vi "PicoScope2000UnitInfoSingle.vi"(8 "error in (no error)":errorcluster, 9 "info Enum":i16(ring), 11 "Handle in":i16) -> (0 "error out":errorcluster, 1 "trimmed string":string, 3 "handle out":i16)   [LabVIEW 2009]
uses:
  ps2000.dll
panel:
  out "status":i16
  out "stringLength":i16
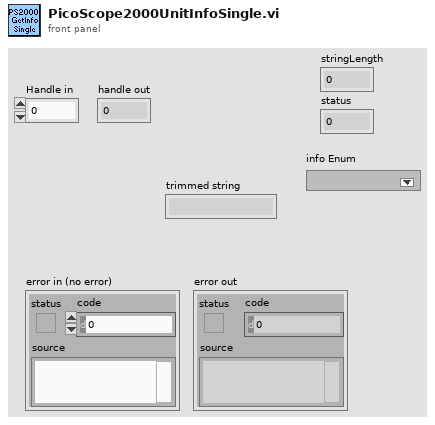
[diagram p1: front panel]
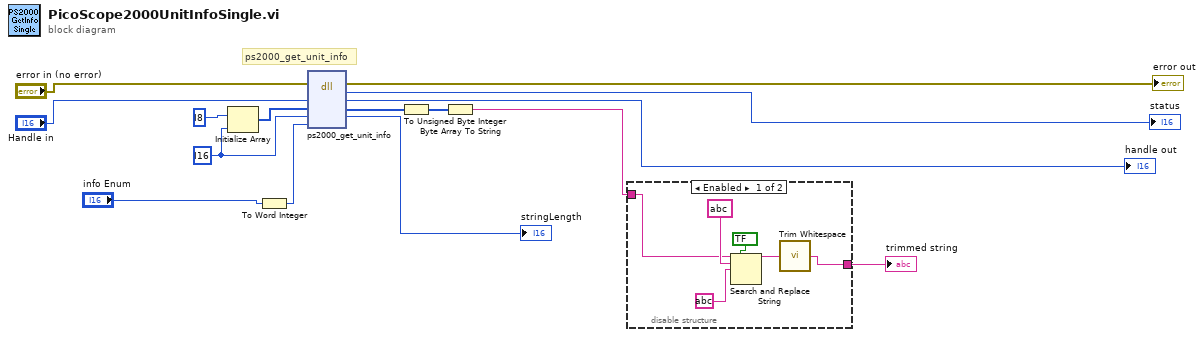
[diagram p0: block diagram]
diagram:
  w11 = i16 ? ("stringLength")
  # "ps2000_get_unit_info"
  n1 = Initialize Array(i8 ? ("element"), w11) -> (w12:i8[])
  n2 = To Word Integer(number="info Enum") -> (16bit integer=w14:i16)
  n3 = dll-call lib="PS2000.dll" fn="ps2000_get_unit_info"(error in="error in (no error)", "handle"="Handle in", "unitInfo"=w12, "stringLength"=w11, "line"=w14) -> (error out=→"error out":errorcluster, "status"=→"status":i16, "handle"=→"handle out":i16, "unitInfo"=w9:i8[], "stringLength"=→"stringLength":i16)  [unwired: 3 in, 1 out]
  n4 = To Unsigned Byte Integer(number=w9) -> (unsigned 8bit integer=w10:u8[])
  n5 = Byte Array To String(unsigned byte array=w10) -> (string=w4:string)
  n6 = disable-structure shown="Enabled" {
    disable-tunnel: w4 -> [w16 w22]
    disable-tunnel: [w17 w22] -> w15
    frame #0 {
      n7 = Search and Replace String(replace all?=bool ? ("replace all? (F)"), input string=w16, search string=string ?, replace string=string ?) -> (result string=w19:string)  [unwired: 4 in, 3 out]
      n8 = call <vilib>:"Trim Whitespace.vi"("string"=w19) -> ("trimmed string"=w17:string)  [unwired: 1 in]
    }
    frame #1 {
    }
  }
  "trimmed string" <- w15
